vi "Drive Distance V2.vi"(8 "Tolerance":dbl=2.0 format="%#_13g", 9 "output range":cluster{"output high":dbl, "output low":dbl}={"output high"=0.55, "output low"=-0.55}, 11 "Distance Set Point":dbl=80.0) -> (3 "Done?":bool)   [LabVIEW 2016]
uses:
  Robot Values.vi
  <vilib>/addons/control/pid/pid.llb/PID (DBL).vi
  <vilib>/addons/control/pid/NI_PID_pid.lvlib
  <vilib>/ptbypt/NI_PtbyPt.lvlib
panel:
  in  "Time Tolerance":dbl=0.15 format="%#_13g"
  out "Elapsed Time (s)":dbl=5.950915813446045
  in  "Error PID gains":T1={"proportional gain (Kc)"=0.1, "integral time (Ti, min)"=0.0, "derivative time (Td, min)"=0.0} {"derivative time (Td, min)" format="%.3f"; "integral time (Ti, min)" format="%.3f"; "proportional gain (Kc)" format="%.3f"}
  in  "PID gains":T1={"proportional gain (Kc)"=0.045, "integral time (Ti, min)"=0.011, "derivative time (Td, min)"=0.0} {"derivative time (Td, min)" format="%.3f"; "integral time (Ti, min)" format="%.3f"; "proportional gain (Kc)" format="%.3f"}
  # "prac:\n.045\n.013\n.0000"
  # "Comp:\n.042\n0\n0"
  # "Comp:\n.045\n.011\n0"
  # "Comp:\n.1\n0\n0"
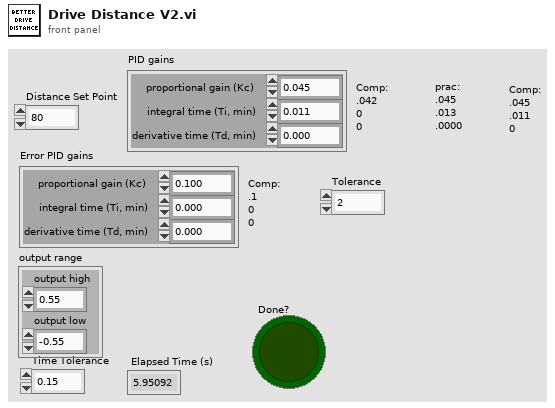
[diagram p1: front panel]
types:
  T1 = cluster{"proportional gain (Kc)":dbl, "integral time (Ti, min)":dbl, "derivative time (Td, min)":dbl}
  T2 = typedef "Robot Values.ctl" = cluster{"Robot Drive":cluster{"Left Motor Power":dbl, "Right Motor Power":dbl, "Left Encoder Value":dbl, "Right Encoder Value":dbl, "High Gear?":bool, "PTO?":bool}, "Sensors":cluster{"Gyro Angle":u16, "Recalibrate Gyro":bool, "Reset Gyro":bool, "Ultrasonic":dbl}, "Shooter":cluster{"Prep Wheels":bool, "Shoot":bool, "Left Shooter Wheel Speed":dbl, "Wheels Moving":bool, "Shooter Prepped":bool, "Shooter RPS SP":dbl, "Shooting?":bool, "Left Shooter Wheel Power":dbl, "Right Shooter Wheel Power":dbl, "Acquisition Conveyor Power":dbl, "Hopper Beater Bar Power":dbl, "Filtered Left Shooter Speed":dbl, "Acquisition Motor Power":dbl, "Joystick Add":dbl, "D-Pad Add":dbl, "Shooter Use PID?":bool}, "Robot States":cluster{"Drive mode":string, "Alliance":T3, "Position":T4}, "Gear":cluster{"Ejection Active":bool}}
  T3 = typedef "WPI_DriverStationAllianceInfo.ctl" = enum16{"Red", "Blue", "Invalid"}
  T4 = typedef "WPI_DriverStationPositionInfo.ctl" = enum16{"1", "2", "3"}
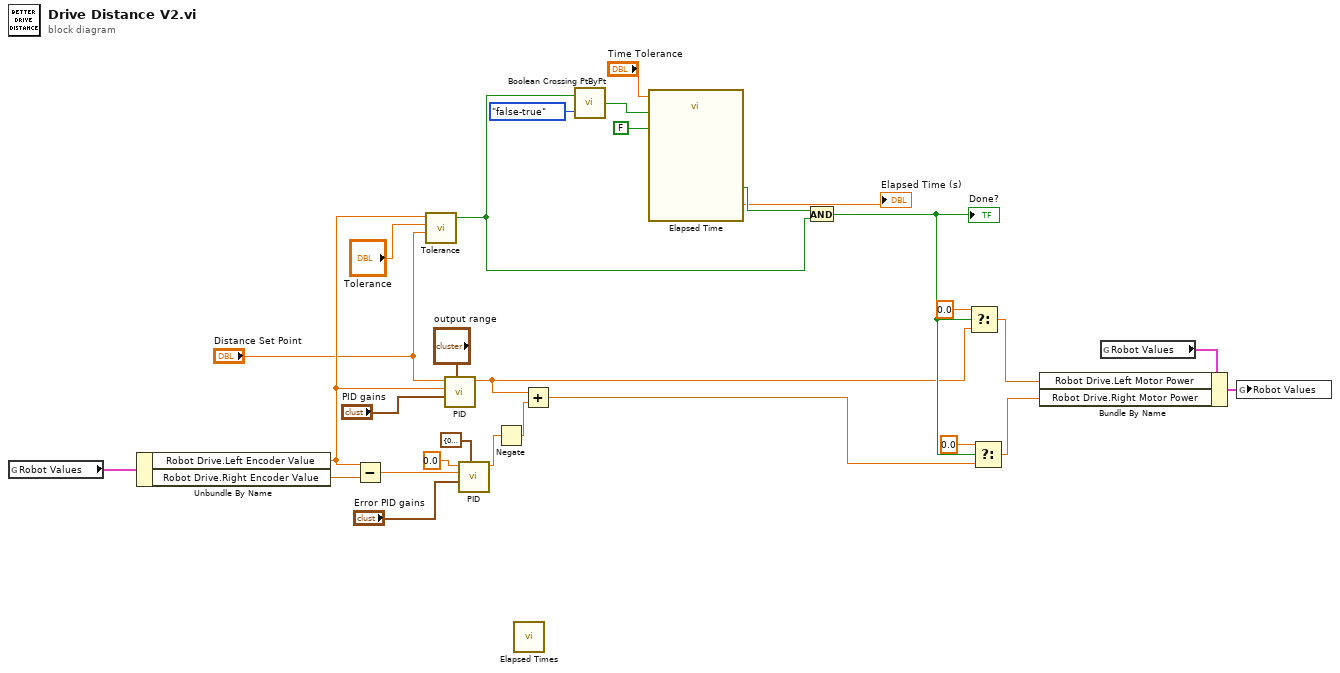
[diagram p0: block diagram]
diagram:
  n1 = global read "Robot Values.vi" "Robot Values"() -> (w29:T2)
  n2 = Unbundle By Name(w29) -> ("Robot Drive.Left Encoder Value"=w17:dbl, "Robot Drive.Right Encoder Value"=w24:dbl)
  n3 = Subtract(x=w17, y=w24) -> (x-y=w23:dbl)
  n4 = call "Tolerance.vi"("Setpoint"="Distance Set Point", "Tolerance"="Tolerance", "Current Value"=w17) -> ("In Range?"=w8:bool)  [unwired: 8 in]
  n5 = call-poly <vilib>:"PID.vi"("output range"="output range", "PID gains"="PID gains", "process variable"=w17, "setpoint"="Distance Set Point") -> ("output"=w4:dbl)  [unwired: 6 in, 1 out]
  n6 = call-poly <vilib>:"PID.vi"("output range"=cluster{"output high":dbl, "output low":dbl} {"output high"=0.55, "output low"=-0.55}, "PID gains"="Error PID gains", "process variable"=w23, "setpoint"=0.0) -> ("output"=w19:dbl)  [unwired: 6 in, 1 out]
  n7 = Negate(x=w19) -> (-x=w18:dbl)
  n8 = call "Elapsed Times.vi"() -> ()  [unwired: 3 in, 1 out]
  n9 = Add(x=w4, y=w18) -> (x+y=w2:dbl)
  n10 = call <vilib>:"Boolean Crossing PtByPt.vi"("direction"=enum16{"either", "false-true", "true-false"}."false-true", "input"=w8) -> ("crossing"=w13:bool)  [unwired: 1 in]
  n11 = call "Elapsed Time"("Time Target (s)"="Time Tolerance", "Reset"=w13, "Auto Reset"=FALSE) -> ("Elapsed Time (s)"=→"Elapsed Time (s)":dbl, "Time has Elapsed"=w10:bool)  [unwired: 9 in, 6 out]
  n12 = And(x=w10, y=w8) -> (x .and. y?=w5:bool)
  "Done?" <- w5
  n13 = Select(t=0.0, s=w5, f=w4) -> (s? t:f=w3:dbl)
  n14 = Select(t=0.0, s=w5, f=w2) -> (s? t:f=w1:dbl)
  n15 = global read "Robot Values.vi" "Robot Values"() -> (w25:T2)
  n16 = Bundle By Name(cluster=w25, "Robot Drive.Left Motor Power"=w3, "Robot Drive.Right Motor Power"=w1) -> (w26:T2)
  n17 = global write "Robot Values.vi" "Robot Values"(w26) -> ()
